vi "enable.vi"(8 "error in (no error)":errorcluster, 10 "model in":refnum<class "IModel.lvclass">, 11 "DisabledState in":refnum<class "DisabledState.lvclass">) -> (0 "error out":errorcluster, 2 "model out":refnum<class "IModel.lvclass">, 3 "DisabledState out":refnum<class "DisabledState.lvclass">)   [LabVIEW 2016, in "States.lvlib" / "DisabledState.lvclass"]
uses:
  DisabledState.lvclass
  IModel/IModel.lvclass
  Typedefs/CommandValue.ctl
  ts_sallv_sedspectrometer/DataTypes/logevent_SummaryState.ctl
  ts_sallv_sedspectrometer/DataTypes/logevent_DetailedState.ctl
  Typedefs/SEDSpectrometerTypedefs.lvlib
  ts_sallv_sedspectrometer/SALLV_sedSpectrometer.lvlib
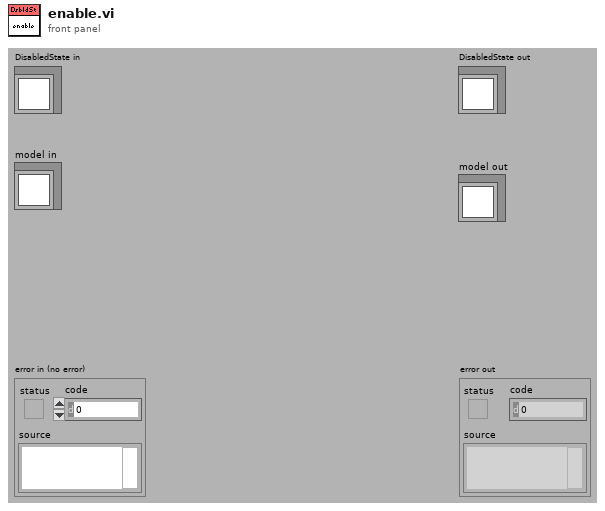
[diagram p1: front panel]
types:
  T1 = typedef "SALLV_sedSpectrometer.lvlib/logevent_DetailedState.ctl" = cluster{"detailedState":enum32{"", "DisabledState", "EnabledState", "FaultState", "OfflineState", "StandbyState", "ImagingState", "NotImagingState"}, "priority":i32}
  T2 = typedef "SALLV_sedSpectrometer.lvlib/logevent_SummaryState.ctl" = cluster{"summaryState":enum32{"", "DisabledState", "EnabledState", "FaultState", "OfflineState", "StandbyState"}, "priority":i32}
  T3 = typedef "SEDSpectrometerTypedefs.lvlib/CommandValue.ctl" = enum16{"clearError", "disable", "enable", "exit", "GoToStandby", "OnHeartbeat", "OnIncomingMessagingError", "OnInterrupt", "start", "captureSpectImage", "setSpectTempSetpoint", "stopImageCapture"}
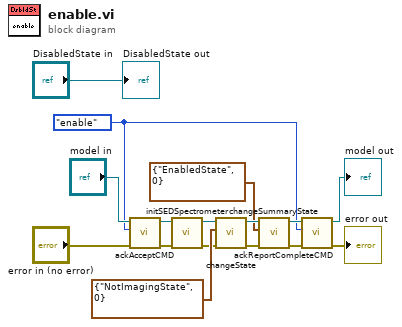
[diagram p0: block diagram]
diagram:
  w7 = CommandValue."enable" ("CommandValue")
  n1 = call-dynamic "ackAcceptCMD.vi"("error in (no error)"="error in (no error)", "CommandValue"=w7, "IModel in"="model in") -> ("error out"=w2:errorcluster, "IModel out"=w4:refnum<class "IModel.lvclass">)  [unwired: 7 in]
  n2 = call-dynamic "initSEDSpectrometer.vi"("error in (no error)"=w2, "IModel in"=w4) -> ("error out"=w1:errorcluster, "IModel out"=w3:refnum<class "IModel.lvclass">)  [unwired: 7 in, 1 out]
  n3 = call-dynamic "changeState.vi"("error in (no error)"=w1, "DetailedState"=T1 {"detailedState"=enum."NotImagingState", "priority"=0} ("logevent_DetailedState"), "IModel in"=w3) -> ("error out"=w14:errorcluster, "IModel out"=w15:refnum<class "IModel.lvclass">)  [unwired: 7 in]
  n4 = call-dynamic "changeSummaryState.vi"("error in (no error)"=w14, "logevent_SummaryState"=T2 {"summaryState"=enum."EnabledState", "priority"=0}, "IModel in"=w15) -> ("error out"=w10:errorcluster, "IModel out"=w9:refnum<class "IModel.lvclass">)  [unwired: 7 in]
  n5 = call-dynamic "ackReportCompleteCMD.vi"("error in (no error)"=w10, "CommandValue"=w7, "IModel in"=w9) -> ("error out"=→"error out":errorcluster, "IModel out"=→"model out":refnum<class "IModel.lvclass">)  [unwired: 7 in]
  "DisabledState out" <- "DisabledState in"
